vi "Configure Trigger (State).vi"(0 "VISA resource name":refnum<visa-resource-name>, 1 "Analog Channel Pattern":string, 2 "Digital Channel Pattern":string, 5 "Clock Source (1: Channel 1)":i32(ring)=1 items=["Channel 1"=1, "Channel 2"=2, "Channel 3"=3, "Channel 4"=4, "Digital 0"=13, "Digital 1"=14, "Digital 2"=15, "Digital 3"=16, "Digital 4"=17, "Digital 5"=18, "Digital 6"=19, "Digital 7"=20, "Digital 8"=21, "Digital 9"=22, "Digital 10"=23, "Digital 11"=24, "Digital 12"=25, "Digital 13"=26, "Digital 14"=27, "Digital 15"=28], 7 "State Condition (0:AND)":u16(ring) items=["AND", "NAND"], 9 "Clock Slope (0: Positive)":u16(ring) items=["Positive", "Negative"], 11 "error in (no error)":errorcluster) -> (4 "VISA resource name out":refnum<visa-resource-name>, 15 "error out":errorcluster)   [LabVIEW 2012, in "Agilent 8000 Series.lvlib"]
doc: "Configures state trigger settings for an oscilloscope. It configures logic pattern to look for, the condition to trigger on, and Clock Slope."
uses:
  <instrlib>/Agilent 8000 Series/Agilent 8000 Series.lvlib
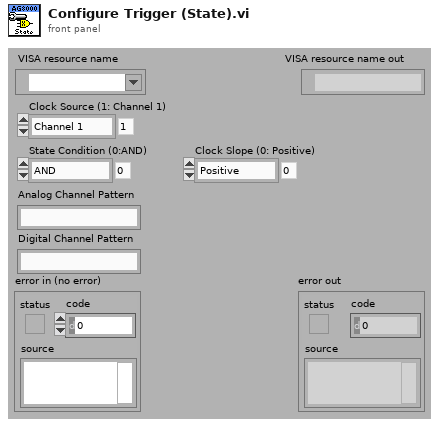
[diagram p1: front panel]
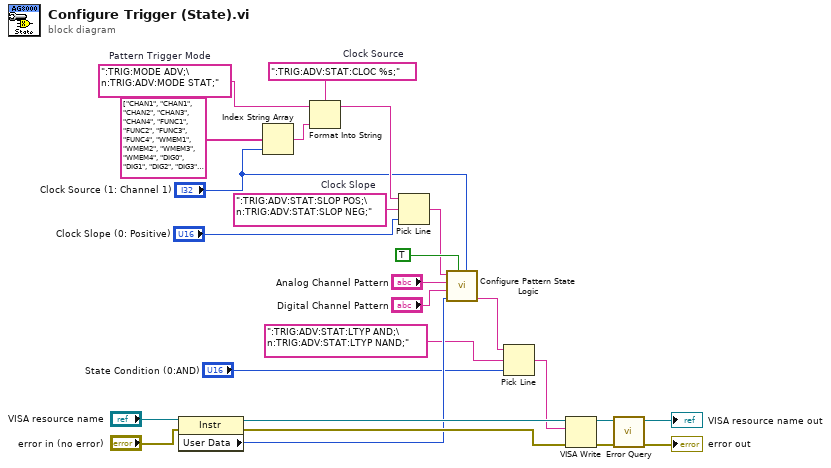
[diagram p0: block diagram]
diagram:
  w8 = ":TRIG:ADV:STAT:SLOP POS;\n:TRIG:ADV:STAT:SLOP NEG;"  # Clock Slope
  w14 = ":TRIG:ADV:STAT:CLOC %s;"  # Clock Source
  w4 = ":TRIG:MODE ADV;\n:TRIG:ADV:MODE STAT;"  # Pattern Trigger Mode
  n1 = property class="Instr"(reference="VISA resource name", error in="error in (no error)") -> (reference out=w18:refnum<visa-resource-name>, error out=w17:errorcluster, "User Data"=w15:u32)
  n2 = Index String Array(1:"Clock Source (1: Channel 1)", 2:string[] ["CHAN1", "CHAN1", "CHAN2", "CHAN3", "CHAN4", "FUNC1", "FUNC2", "FUNC3", "FUNC4", "WMEM1", "WMEM2", "WMEM3", "WMEM4", "DIG0", "DIG1", "DIG2", "DIG3", "DIG4", "DIG5", "DIG6", "DIG7", "DIG8", "DIG9", "DIG10", "DIG11", "DIG12", "DIG13", "DIG14", "DIG15", "AUX", "LINE", "DONT"]) -> (0:w9:string)  [unwired: 1 in]
  n3 = Format Into String(format string=w14, initial string=w4, w9) -> (resulting string=w6:string)  [unwired: 1 in, 1 out]
  n4 = Pick Line(string ("")=w6, multi-line string=w8, line index="Clock Slope (0: Positive)") -> (output string=w3:string)
  n5 = call "Configure Pattern State Logic.vi"("Clock Source (1: Channel 1)"="Clock Source (1: Channel 1)", "Enable Clock Source (False)"=TRUE ("Enable Clock Source (True)"), "Model"=w15, "Digital Channel Pattern"="Digital Channel Pattern", "Analog Channel Pattern"="Analog Channel Pattern", "Input"=w3) -> ("Output"=w1:string)  [unwired: 5 in]
  n6 = Pick Line(string ("")=w1, multi-line string=":TRIG:ADV:STAT:LTYP AND;\n:TRIG:ADV:STAT:LTYP NAND;", line index="State Condition (0:AND)") -> (output string=w11:string)
  n7 = VISA Write(VISA resource name=w18, write buffer=w11, error in (no error)=w17) -> (VISA resource name out=w23:refnum<visa-resource-name>, error out=w22:errorcluster)  [unwired: 1 out]
  n8 = call <instrlib>:"Error Query.vi"("error in (no error)"=w22, "VISA resource name"=w23) -> ("error out"=→"error out":errorcluster, "VISA resource name out"=→"VISA resource name out":refnum<visa-resource-name>)  [unwired: 6 in, 2 out]
